vi "Temperature Warnings.vi"(8 "Error In":errorcluster, 11 "Weather Data In":T1={"Current Temperature"=0.0, "Max Temperature"=0.0, "Min Temperature"=0.0, "Warning?"=FALSE, "Warning Text"="No Warning"}) -> (0 "Error Out":errorcluster, 3 "Weather Data Out":T1={"Current Temperature"=0.0, "Max Temperature"=0.0, "Min Temperature"=0.0, "Warning?"=FALSE, "Warning Text"="No Warning"})   [LabVIEW 2015]
doc: "In this exercise, you develop an icon and a connector pane for this subVI then test calling the subVI from a calling VI."
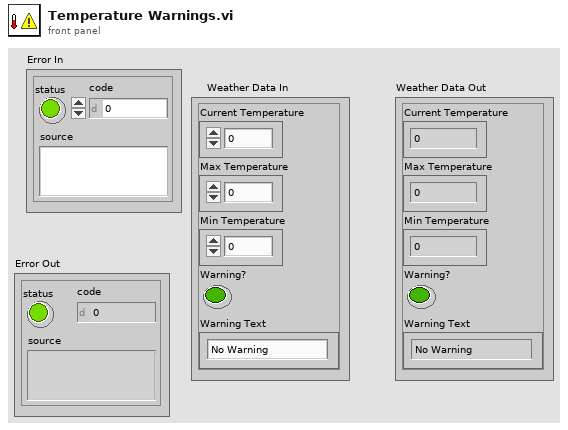
[diagram p1: front panel]
types:
  T1 = cluster{"Current Temperature":dbl, "Max Temperature":dbl, "Min Temperature":dbl, "Warning?":bool, "Warning Text":string}
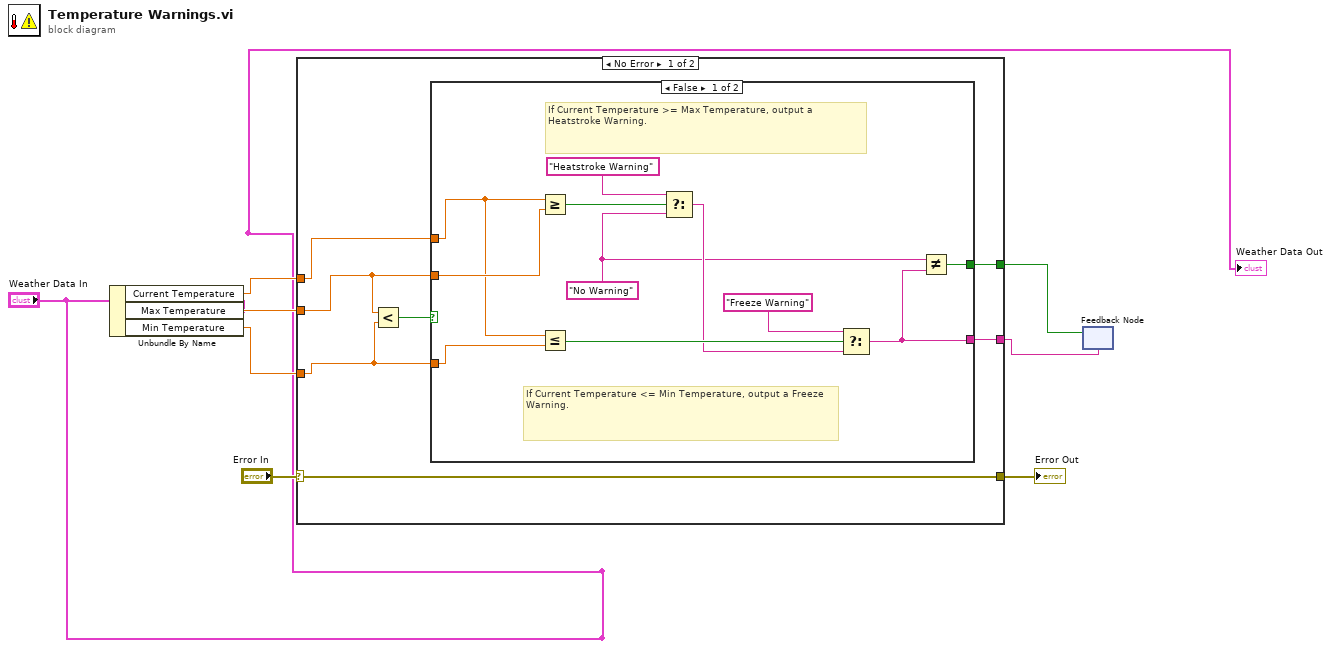
[diagram p0: block diagram]
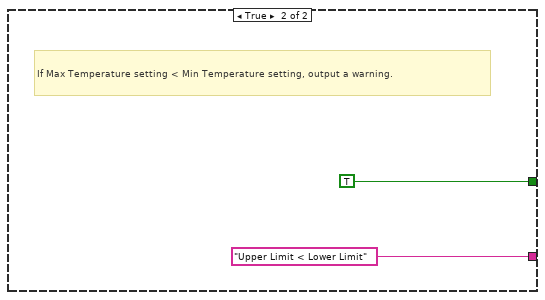
[diagram p2: hidden frame]
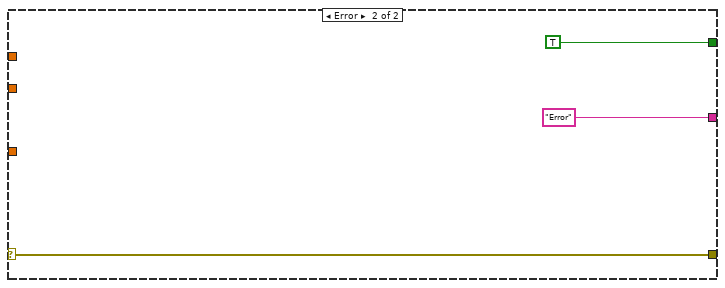
[diagram p3: hidden frame]
diagram:
  n1 = Unbundle By Name("Weather Data In") -> ("Current Temperature"=w6:dbl, "Max Temperature"=w5:dbl, "Min Temperature"=w4:dbl)
  n2 = case shown="No Error" "Error In" {
    selector: "Error In" -> [w14 w31]
    tunnel: [w15 "Error" ("f")] -> w1
    tunnel: [w9 TRUE] -> w2
    tunnel: [w14 w31] -> w7
    tunnel: w6 -> [w12 _]
    tunnel: w5 -> [w11 _]
    tunnel: w4 -> [w10 _]
    frame No Error {
      n3 = Less?(x=w11, y=w10) -> (x < y?=w13:bool)
      n4 = case shown="False" w13 {
        tunnel: [w20 "Upper Limit < Lower Limit" ("f")] -> w15
        tunnel: [w16 TRUE] -> w9
        tunnel: w12 -> [w17 _]
        tunnel: w11 -> [w19 _]
        tunnel: w10 -> [w18 _]
        frame False {
          w21 = "No Warning" ("f")
          # "If Current Temperature >= Max Temperature, output a Heatstroke Warning."
          # "If Current Temperature <= Min Temperature, output a Freeze Warning."
          n5 = Greater Or Equal?(x=w17, y=w19) -> (x >= y?=w26:bool)
          n6 = Less Or Equal?(x=w17, y=w18) -> (x <= y?=w23:bool)
          n7 = Select(t="Heatstroke Warning", s=w26, f=w21) -> (s? t:f=w22:string)
          n8 = Select(t="Freeze Warning", s=w23, f=w22) -> (s? t:f=w20:string)
          n9 = Not Equal?(x=w21, y=w20) -> (x != y?=w16:bool)
        }
        frame True {
          # "If Max Temperature setting < Min Temperature setting, output a warning."
        }
      }
    }
    frame Error {
    }
  }
  "Error Out" <- w7
  n10 = feedback-in #1(w2) -> ()
  n11 = feedback #1(w1) -> ()  [unwired: 1 in]
  "Weather Data Out" <- "Weather Data In"
